vi "扫BOXID.vi"(8 "error in (no error)":errorcluster caption="错误输入（无错误）", 11 "超时秒数":dbl) -> (0 "error out":errorcluster caption="错误输出", 2 "BOXID":string, 3 "result":bool)   [LabVIEW 2017]
uses:
  <vilib>/Instr/_visa.llb/VISA Configure Serial Port (Instr).vi
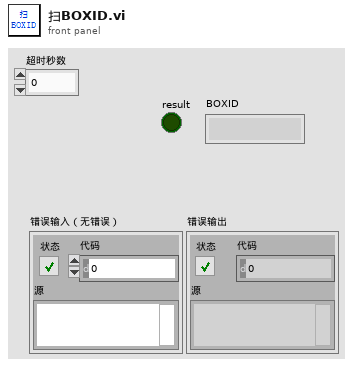
[diagram p1: front panel]
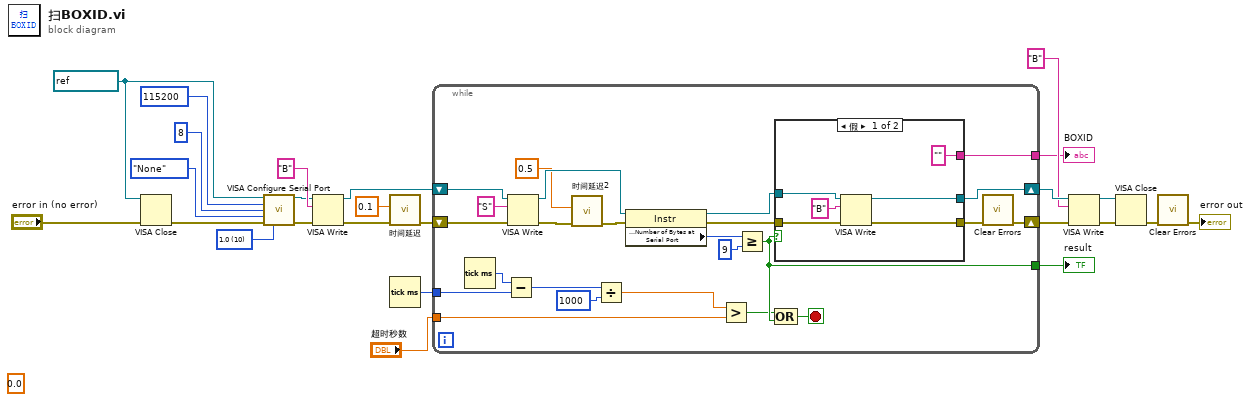
[diagram p0: block diagram]
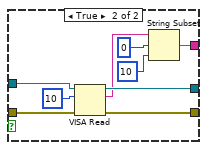
[diagram p2: hidden frame]
diagram:
  (unwired) 0.0 ("默认(0 DBL)")
  w19 = u16 10 items=["1.0"=10, "1.5"=15, "2.0"=20] ("stop bits (10: 1 bit)")
  w18 = refnum<visa-resource-name> "COM1" ("VISA resource name")
  n1 = VISA Close(VISA resource name=w18, error in (no error)="error in (no error)") -> (error out=w17:errorcluster)
  n2 = call-poly "VISA Configure Serial Port"("VISA resource name"=w18, "baud rate (9600)"=u32 115200, "data bits (8)"=u16 8, "parity (0:none)"=enum16{"None", "Odd", "Even", "Mark", "Space"}."None", "error in (no error)"=w17, "stop bits (10: 1 bit)"=w19) -> ("VISA resource name out"=w14:refnum<visa-resource-name>, "error out"=w15:errorcluster)  [unwired: 8 in]
  n3 = VISA Write(VISA resource name=w14, write buffer="B" ("写入缓冲区"), error in (no error)=w15) -> (VISA resource name out=w13:refnum<visa-resource-name>, error out=w12:errorcluster)  [unwired: 1 out]
  n4 = call "时间延迟"("error in (no error)"=w12, "Delay Time (s)"=0.1) -> ("error out"=w11:errorcluster)  [unwired: 9 in]
  n5 = Tick Count (ms)() -> (millisecond timer value=w2:u32)
  n6 = while {
    tunnel: [w45] -> w6
    tunnel: [w44] -> w3
    shift-right: [w49] -> w24
    shift-left: w13 -> [w47]
    shift-right: [w48] -> w23
    shift-left: w11 -> [w46]
    tunnel: w2 -> [w30]
    tunnel: "超时秒数" -> [w26]
    stop <- w43 stop-if-true
    n7 = Tick Count (ms)() -> (millisecond timer value=w31:u32)
    n8 = Subtract(x=w31, y=w30) -> (x-y=w29:u32)
    n9 = VISA Write(VISA resource name=w47, write buffer="S" ("写入缓冲区"), error in (no error)=w46) -> (VISA resource name out=w40:refnum<visa-resource-name>, error out=w35:errorcluster)  [unwired: 1 out]
    n10 = call "时间延迟2"("error in (no error)"=w35, "Delay Time (s)"=0.5) -> ("error out"=w34:errorcluster)  [unwired: 9 in]
    n11 = Divide(x=w29, y=u32 1000) -> (x/y=w27:dbl)
    n12 = property class="Instr"(reference=w40, error in=w34) -> (reference out=w39:refnum<visa-resource-name>, error out=w33:errorcluster, "Serial Settings:Number of Bytes at Serial Port"=w38:u32)
    n13 = Greater?(x=w27, y=w26) -> (0:w42:bool)
    n14 = Greater Or Equal?(x=w38, y=u32 9) -> (x >= y?=w44:bool)
    n15 = case shown="假" w44 {
      tunnel: [w52 w64] -> w49
      tunnel: w39 -> [w54 w63]
      tunnel: w33 -> [w53 w62]
      tunnel: ["" ("read buffer") w61] -> w45
      tunnel: [w51 w56] -> w36
      frame False {
        n16 = VISA Write(VISA resource name=w54, write buffer="B" ("写入缓冲区"), error in (no error)=w53) -> (VISA resource name out=w52:refnum<visa-resource-name>, error out=w51:errorcluster)  [unwired: 1 out]
      }
      frame True {
        n17 = VISA Read(VISA resource name=w63, byte count=u32 10 ("字节总数"), error in (no error)=w62) -> (VISA resource name out=w64:refnum<visa-resource-name>, read buffer=w60:string, error out=w56:errorcluster)  [unwired: 1 out]
        n18 = String Subset(string=w60, offset (0)=0, length (rest)=10 ("length (rest)")) -> (substring=w61:string)
      }
    }
    n19 = Compound Arithmetic op=OR(w42, w44) -> (w43:bool)
    n20 = call <vilib>:"Clear Errors.vi"("error in (no error)"=w36) -> ("error out"=w48:errorcluster)  [unwired: 5 in, 1 out]
  }
  "result" <- w3
  "BOXID" <- w6
  n21 = VISA Write(VISA resource name=w24, write buffer="B" ("写入缓冲区"), error in (no error)=w23) -> (VISA resource name out=w8:refnum<visa-resource-name>, error out=w9:errorcluster)  [unwired: 1 out]
  n22 = VISA Close(VISA resource name=w8, error in (no error)=w9) -> (error out=w5:errorcluster)
  n23 = call <vilib>:"Clear Errors.vi"("error in (no error)"=w5) -> ("error out"=→"error out":errorcluster)  [unwired: 5 in, 1 out]
